vi "FlatToRichnixnet_grpc_ReadSignalWaveformRequest.vi"(5 "OutputClusterType":T1, 11 "InputCluster":T3) -> (3 "OutputCluster":T1)   [LabVIEW 2025, in "grpc-xnet_client.lvlib"]
uses:
  nixnet_grpc_ReadSignalWaveformRequest_Flat.ctl
  nidevice_grpc_Session_Flat.ctl
  nixnet_grpc_TimeOut.ctl
  nixnet_grpc_ReadSignalWaveformRequest.ctl
  nixnet_grpc_ReadSignalWaveformRequest_timeout_enum/nixnet_grpc_ReadSignalWaveformRequest_timeout_enum.lvclass
  nidevice_grpc_Session.ctl
  grpc-xnet_client.lvlib
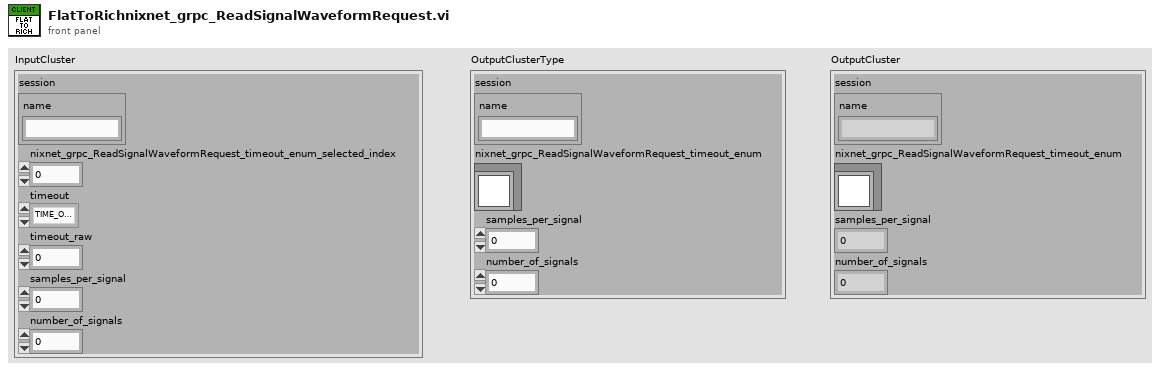
[diagram p1: front panel]
types:
  T1 = typedef "grpc-xnet_client.lvlib/nixnet_grpc_ReadSignalWaveformRequest.ctl" = cluster{"session":T2, "nixnet_grpc_ReadSignalWaveformRequest_timeout_enum":refnum<class "nixnet_grpc_ReadSignalWaveformRequest_timeout_enum.lvclass">, "samples_per_signal":u32, "number_of_signals":u32}
  T2 = typedef "grpc-xnet_client.lvlib/nidevice_grpc_Session.ctl" = cluster{"name":string}
  T3 = typedef "grpc-xnet_client.lvlib/nixnet_grpc_ReadSignalWaveformRequest_Flat.ctl" = cluster{"session":T4, "nixnet_grpc_ReadSignalWaveformRequest_timeout_enum_selected_index":i32, "timeout":T5, "timeout_raw":dbl, "samples_per_signal":u32, "number_of_signals":u32}
  T4 = typedef "grpc-xnet_client.lvlib/nidevice_grpc_Session_Flat.ctl" = cluster{"name":string}
  T5 = typedef "grpc-xnet_client.lvlib/nixnet_grpc_TimeOut.ctl" = enum32{"TIME_OUT_NONE", "TIME_OUT_INFINITE"}
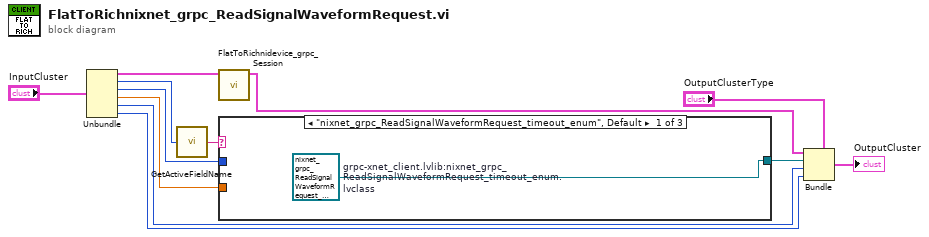
[diagram p0: block diagram]
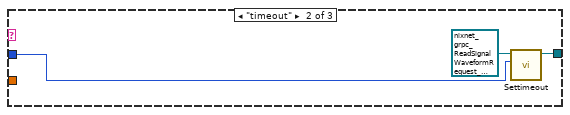
[diagram p2: hidden frame]
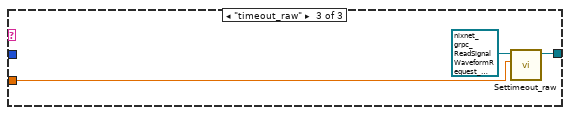
[diagram p3: hidden frame]
diagram:
  n1 = Unbundle "Unbundle"("InputCluster") -> ("session"=w9:T4, "nixnet_grpc_ReadSignalWaveformRequest_timeout_enum_selected_index"=w7:i32, "timeout"=w4:T5, "timeout_raw"=w3:dbl, "samples_per_signal"=w2:u32, "number_of_signals"=w1:u32)
  n2 = call "GetActiveFieldName.vi"("protobuf index"=w7) -> ("oneof field name"=w6:string)
  n3 = call "FlatToRichnidevice_grpc_Session.vi"("InputCluster"=w9) -> ("OutputCluster"=w8:T2)  [unwired: 10 in]
  n4 = case "nixnet_grpc_ReadSignalWaveformRequest_timeout_enum" shown="\"nixnet_grpc_ReadSignalWaveformRequest_timeout_enum\", Default" w6 {
    tunnel: [w13 w15 w18] -> w5
    tunnel: w4 -> [_ w16 _]
    tunnel: w3 -> [_ _ w19]
    frame "nixnet_grpc_ReadSignalWaveformRequest_timeout_enum", Default {
      w13 = refnum<class "nixnet_grpc_ReadSignalWaveformRequest_timeout_enum.lvclass"> refnum  # grpc-xnet_client.lvlib:nixnet_grpc_ReadSignalWaveformRequest_timeout_enum.lvclass
    }
    frame "timeout" {
      n5 = call "Settimeout.vi"("Set_Val"=w16, "OneOfTemplate in"=refnum<class "nixnet_grpc_ReadSignalWaveformRequest_timeout_enum.lvclass"> refnum) -> ("OneOfTemplate out"=w15:refnum<class "nixnet_grpc_ReadSignalWaveformRequest_timeout_enum.lvclass">)  [unwired: 8 in, 1 out]
    }
    frame "timeout_raw" {
      n6 = call "Settimeout_raw.vi"("Set_Val"=w19, "OneOfTemplate in"=refnum<class "nixnet_grpc_ReadSignalWaveformRequest_timeout_enum.lvclass"> refnum) -> ("OneOfTemplate out"=w18:refnum<class "nixnet_grpc_ReadSignalWaveformRequest_timeout_enum.lvclass">)  [unwired: 8 in, 1 out]
    }
  }
  n7 = Bundle "Bundle"(cluster="OutputClusterType", "session"=w8, "nixnet_grpc_ReadSignalWaveformRequest_timeout_enum"=w5, "samples_per_signal"=w2, "number_of_signals"=w1) -> (→"OutputCluster":T1)
